vi "set task trigger.vi"(8 "error in (no error)":errorcluster, 11 "Waveform in":refnum<class "Waveform.lvclass">) -> (0 "error out":errorcluster, 3 "Waveform out":refnum<class "Waveform.lvclass">)   [LabVIEW 2012, in "Waveform.lvclass"]
uses:
  Waveform.lvclass
  <resource>/objmgr/daqmx.rc
  <vilib>/DAQmx/configure/trigger.llb/DAQmx Start Trigger (Digital Edge).vi
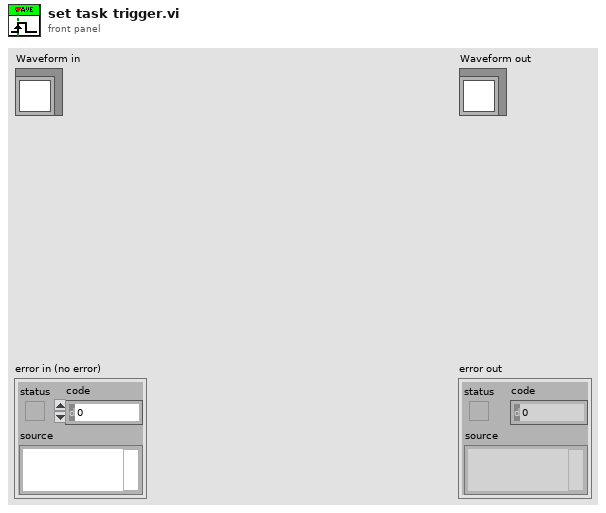
[diagram p1: front panel]
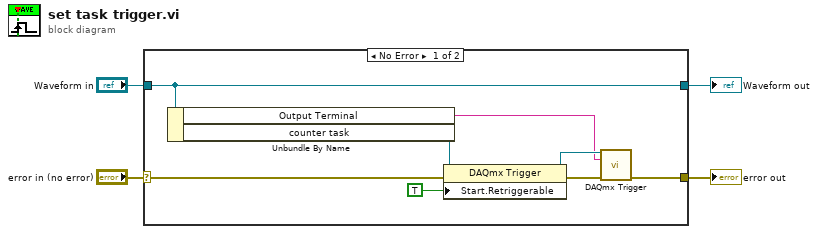
[diagram p0: block diagram]
diagram:
  n1 = case shown="No Error" "error in (no error)" {
    selector: "error in (no error)" -> [w12 w14]
    tunnel: [w6 w14] -> w3
    tunnel: [w5 w13] -> w1
    tunnel: "Waveform in" -> [w5 w13]
    frame No Error {
      n2 = Unbundle By Name(w5) -> ("Output Terminal"=w8:tag, "counter task"=w7:refnum<k21>)
      n3 = property class="DAQmx Trigger"(reference=w7, error in=w12, "Start.Retriggerable"=TRUE) -> (reference out=w9:refnum<k21>, error out=w10:errorcluster)
      n4 = call-poly <vilib>:"DAQmx Trigger.vi"("task/channels in"=w9, "source"=w8, "error in"=w10) -> ("error out"=w6:errorcluster)  [unwired: 11 in, 1 out]
    }
    frame Error {
    }
  }
  "error out" <- w3
  "Waveform out" <- w1
